vi "GetInstReading.vi"(1 "Inst number":string, 2 "Array":cluster{"Inst #":string, "Value":dbl}[](array[cluster])) -> (0 "Reading":dbl)   [LabVIEW 2020]
panel:
  # "When given a cluster array of instrument number/reading pairs,\nreturns the reading of the given instrument"
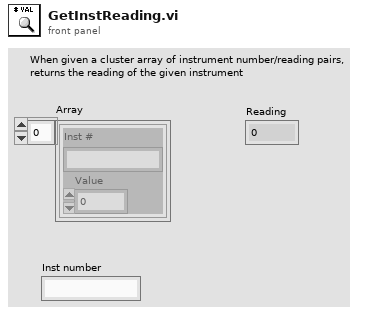
[diagram p1: front panel]
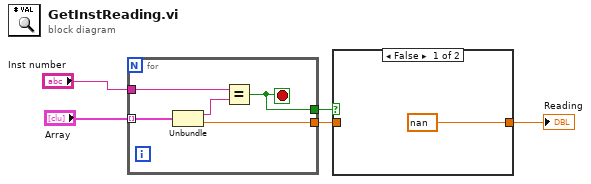
[diagram p0: block diagram]
diagram:
  n1 = for {
    tunnel: "Inst number" -> [w7]
    tunnel: "Array" -> [w10] mode=indexing
    tunnel: [w9] -> w2
    tunnel: [w6] -> w3
    stop <- w6 stop-if-true
    n2 = Unbundle(w10) -> ("Inst #"=w8:string, "Value"=w9:dbl)
    n3 = Equal?(x=w7, y=w8) -> (x = y?=w6:bool)
  }
  n4 = case shown="False" w3 {
    tunnel: w2 -> [_ w12]
    tunnel: [nan w12] -> w1
    frame False {
    }
    frame True {
    }
  }
  "Reading" <- w1
